vi "Test API.vi"() -> ()   [LabVIEW 2020]
uses:
  Add.lvlib
panel:
  out "Result":dbl
  in  "Y":dbl
  in  "X":dbl
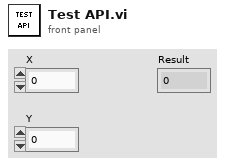
[diagram p1: front panel]
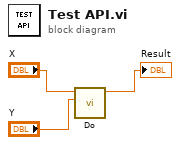
[diagram p0: block diagram]
diagram:
  n1 = call "Do.vi"("Y"="Y", "X"="X") -> ("Result"=→"Result":dbl)  [unwired: 9 in]
